vi "Property Tree_Populate Trees.vi"(4 "Close Items":bool, 5 "VI Ref":refnum<vi>, 6 "Filter":string, 7 "Action":T3, 8 "Error In":errorcluster, 9 "Tree Refs":refnum<vi>[](array[refnum]), 10 "Show":T1, 11 "Properties for Tree In":T2(array[cluster])) -> (0 "error out":errorcluster)   [LabVIEW 2023]
uses:
  controls/action enum.ctl
panel:
  out "exe time (ms)":u32
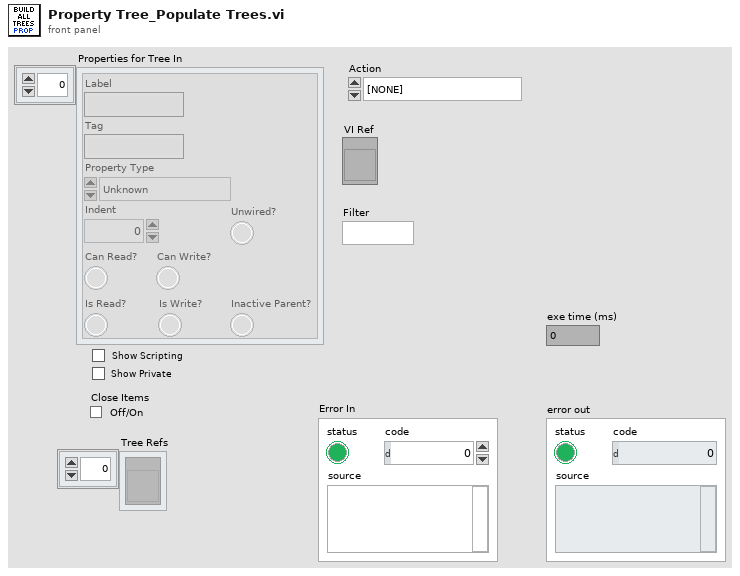
[diagram p1: front panel]
types:
  T1 = cluster{"Show Scripting":bool, "Show Private":bool}
  T2 = cluster{"Label":string, "Tag":string, "Property Type":enum16{"Unknown", "Base", "Scripting", "Private", "Deprecated", "None", "Divider"}, "Indent":u16, "Can Read?":bool, "Can Write?":bool, "Is Read?":bool, "Is Write?":bool, "Inactive Parent?":bool, "Unwired?":bool}[]
  T3 = typedef "action enum.ctl" = enum16{"[NONE]", "Wire Bundle", "Wire Unbundle", "Terminal Unbundle", "Terminal Bundle", "Bundler Move Up", "Bundler Move Down", "Bundler Insert", "Bundler Remove", "Bundler Remove Unwired", "Bundler Rearrange", "In Place Insert", "In Place Remove", "In Place Remove Unwired", "In Place Rearrange", "Wire Properties", "Wire Method", "Terminal Properties", "Terminal Method", "Property Move Up", "Property Move Down", "Properties Insert", "Properties Remove", "Properties Remove Unwired", "Properties Rearrange", "Method Change", "Class for Constant", "Class For Control", "Class For Node", "Class Name to Clipboard"}
  T4 = cluster{"Show":cluster{"Show Scripting":bool, "Show Private":bool}, "Filter":string}
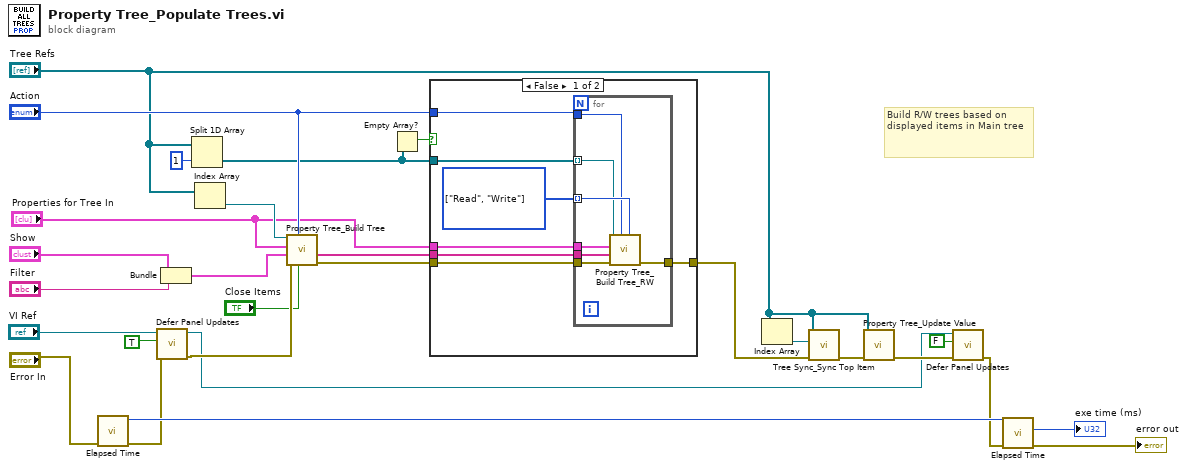
[diagram p0: block diagram]
diagram:
  # "Build R/W trees based on displayed items in Main tree"
  n1 = call "Elapsed Time.vi"("error in"="Error In") -> ("error out"=w5:errorcluster, "millisecond timer value"=w22:u32)  [unwired: 6 in, 3 out]
  n2 = call "Defer Panel Updates.vi"("error in (no error)"=w5, "Defer Panel Updates [T]"=TRUE, "VI Ref"="VI Ref") -> ("error out"=w27:errorcluster, "VI Ref Out"=w23:refnum<vi>)  [unwired: 7 in]
  n3 = Bundle("Show"="Show", "Filter"="Filter") -> (w18:T4)  [unwired: 1 in]
  n4 = Split 1D Array(array="Tree Refs", index=1) -> (second subarray=w11:refnum<vi>[])  [unwired: 1 out]
  n5 = Index Array(array="Tree Refs") -> (element=w12:refnum<vi>)  [unwired: 1 in]
  n6 = call "Property Tree_Build Tree.vi"("Close Items"="Close Items", "Action"="Action", "error in"=w27, "Filter"=w18, "Properties for Tree"="Properties for Tree In", "Tree Ref"=w12) -> ("error out"=w15:errorcluster, "Displayed Items"=w16:string[])  [unwired: 2 in, 2 out]
  n7 = Empty Array?(array=w11) -> (empty?=w10:bool)
  n8 = case shown="False" w10 {
    tunnel: w16 -> [w35 _]
    tunnel: w15 -> [w34 w43]
    tunnel: [w33 w43] -> w4
    tunnel: "Properties for Tree In" -> [w32 _]
    tunnel: "Action" -> [w30 _]
    tunnel: w11 -> [w29 _]
    frame False {
      w31 = enum16{"Main", "Write", "Read"}[] [enum."Read", enum."Write"] items=["Main", "Write", "Read"] ("Tree Type")
      n9 = for {
        tunnel: w35 -> [w42]
        tunnel: w32 -> [w39]
        tunnel: w34 -> [w41]
        tunnel: [w40] -> w33
        tunnel: w31 -> [w38] mode=indexing
        tunnel: w30 -> [w37]
        tunnel: w29 -> [w36] mode=indexing
        n10 = call "Property Tree_Build Tree_RW.vi"("Tree Type"=w38, "Action"=w37, "error in"=w41, "Displayed Items"=w42, "Properties for Tree"=w39, "Tree Ref"=w36) -> ("error out"=w40:errorcluster)  [unwired: 3 in, 2 out]
      }
    }
    frame True {
    }
  }
  n11 = Index Array(array="Tree Refs") -> (element=w1:refnum<vi>)  [unwired: 1 in]
  n12 = call "Tree Sync_Sync Top Item.vi"("error in"=w4, "Changed Tree Control Ref"=w1, "All Tree Control Refs"="Tree Refs") -> ("error out"=w3:errorcluster)  [unwired: 8 in]
  n13 = call "Property Tree_Update Value.vi"("error in"=w3, "Tree Ref Array Out"="Tree Refs") -> ("error out"=w25:errorcluster)  [unwired: 9 in]
  n14 = call "Defer Panel Updates.vi"("error in (no error)"=w25, "Defer Panel Updates [T]"=FALSE, "VI Ref"=w23) -> ("error out"=w8:errorcluster)  [unwired: 7 in, 1 out]
  n15 = call "Elapsed Time.vi"("error in"=w8, "past time"=w22) -> ("error out"=→"error out":errorcluster, "elapsed time (ms)"=→"exe time (ms)":u32)  [unwired: 5 in, 3 out]
